vi "Configure Measurement.vi"(0 "VISA resource name":refnum<visa-resource-name>, 1 "Channel (1: Channel 1)":u16(ring)=1 items=["Channel 1"=1, "Channel 2"=2], 2 "Integration Time (4: 10 NPLCs)":u16(ring)=4 format="%.0g" items=["0.02 NPLC", "0.2 NPLC", "1 NPLC", "2 NPLCs", "10 NPLCs", "20 NPLCs", "100 NPLCs", "200 NPLCs"], 5 "Function (0: DC Volts)":u16(ring) items=["DC Volts", "DC Voltage Ratio", "DC Voltage Difference", "2 Wire Resistance", "4 Wire Resistance", "Temperature"], 7 "Auto Range (T:Enable)":bool=TRUE, 9 "Enable Offset Compensation (F: Disable)":bool, 11 "error in (no error)":errorcluster, 12 "Manual Range (0.001)":dbl=0.001, 13 "Resolution (1E-9)":dbl=1e-09 format="%^#_6g") -> (4 "VISA resource name out":refnum<visa-resource-name>, 15 "error out":errorcluster)   [LabVIEW 2022 SP3, in "Agilent 34420.lvlib"]
doc: "Configures the measurement type, resolution, and range on the instrument.\n\n<B>Note:</B>\n\nFor temperature measurements, further configuration is required. <B>Configure Temperature</B> VI should be called after this VI."
uses:
  Agilent 34420.lvlib
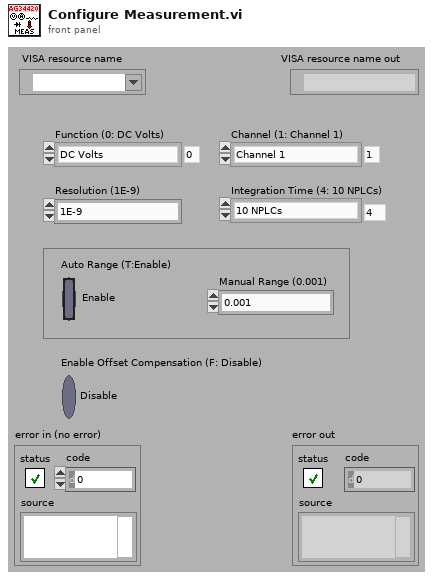
[diagram p1: front panel]
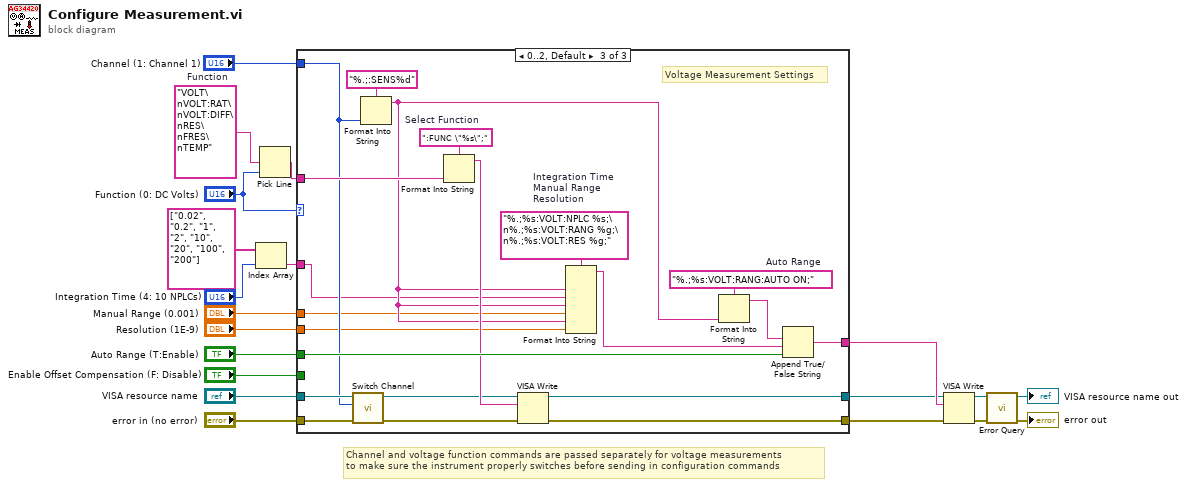
[diagram p0: block diagram]
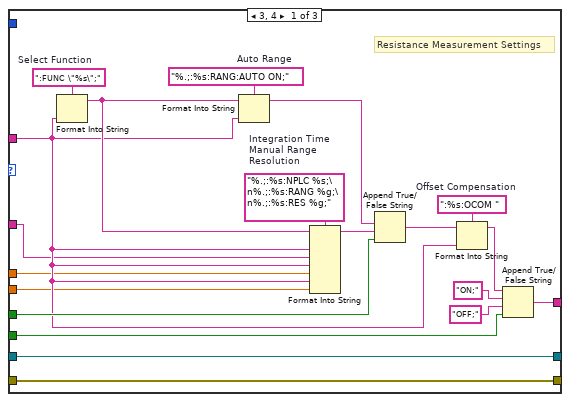
[diagram p2: hidden frame]
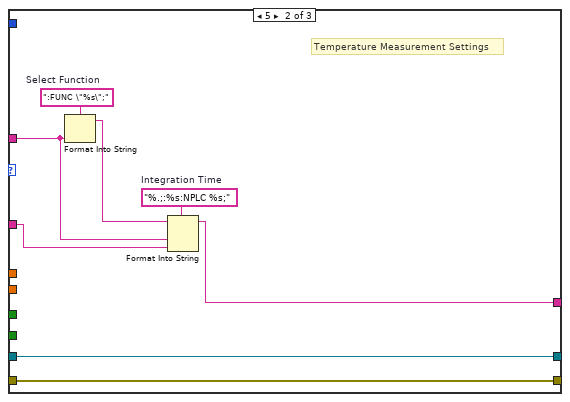
[diagram p3: hidden frame]
diagram:
  w18 = "VOLT\nVOLT:RAT\nVOLT:DIFF\nRES\nFRES\nTEMP"  # Function
  # "Channel and voltage function commands are passed separately for voltage measurements\nto make sure the instrument properly switches before sending in configuration commands"
  n1 = Index Array(array=string[] ["0.02", "0.2", "1", "2", "10", "20", "100", "200"], index="Integration Time (4: 10 NPLCs)") -> (element=w3:string)
  n2 = Pick Line(multi-line string=w18, line index="Function (0: DC Volts)") -> (output string=w15:string)  [unwired: 1 in]
  n3 = case shown="0..2, Default" "Function (0: DC Volts)" {
    tunnel: w15 -> [w24 w42 w65]
    tunnel: "Auto Range (T:Enable)" -> [w26 _ w64]
    tunnel: [w27 w48 w62] -> w13
    tunnel: "VISA resource name" -> [w29 w47 w61]
    tunnel: "error in (no error)" -> [w28 w46 w60]
    tunnel: "Channel (1: Channel 1)" -> [_ _ w59]
    tunnel: [w29 w47 w55] -> w9
    tunnel: [w28 w46 w54] -> w8
    tunnel: "Enable Offset Compensation (F: Disable)" -> [w25 _ _]
    tunnel: "Resolution (1E-9)" -> [w23 _ w50]
    tunnel: "Manual Range (0.001)" -> [w22 _ w51]
    tunnel: w3 -> [w21 w41 w49]
    frame 3, 4 {
      w34 = "%.;:%s:RANG:AUTO ON;"  # Auto Range
      w32 = "%.;:%s:NPLC %s;\n%.;:%s:RANG %g;\n%.;:%s:RES %g;"  # Integration Time Manual Range Resolution
      w31 = ":%s:OCOM "  # Offset Compensation
      w30 = ":FUNC \"%s\";"  # Select Function
      # "Resistance Measurement Settings"
      n4 = Format Into String(format string=w30, w24) -> (resulting string=w36:string)  [unwired: 2 in, 1 out]
      n5 = Format Into String(format string=w34, initial string=w36, w24) -> (resulting string=w35:string)  [unwired: 1 in, 1 out]
      n6 = Format Into String(format string=w32, initial string=w36, w24, w21, w24, w22, w24, w23) -> (resulting string=w33:string)  [unwired: 1 in, 1 out]
      n7 = Append True/False String(1:w26, 2:w33, 3:w35) -> (0:w37:string)  [unwired: 1 in]
      n8 = Format Into String(format string=w31, initial string=w37, w24) -> (resulting string=w38:string)  [unwired: 1 in, 1 out]
      n9 = Append True/False String(1:w25, 2:"OFF;" ("false string"), 3:"ON;" ("true string"), 4:w38) -> (0:w27:string)
    }
    frame 5 {
      w44 = ":FUNC \"%s\";"  # Select Function
      w45 = "%.;:%s:NPLC %s;"  # Integration Time
      # "Temperature Measurement Settings"
      n10 = Format Into String(format string=w44, w42) -> (resulting string=w43:string)  [unwired: 2 in, 1 out]
      n11 = Format Into String(format string=w45, initial string=w43, w42, w41) -> (resulting string=w48:string)  [unwired: 1 in, 1 out]
    }
    frame 0..2, Default {
      w67 = "%.;%s:VOLT:RANG:AUTO ON;"  # Auto Range
      w68 = "%.;%s:VOLT:NPLC %s;\n%.;%s:VOLT:RANG %g;\n%.;%s:VOLT:RES %g;"  # Integration Time Manual Range Resolution
      w69 = ":FUNC \"%s\";"  # Select Function
      # "Voltage Measurement Settings"
      n12 = call "Switch Channel.vi"("error in (no error)"=w60, "Channel (1: Channel 1)"=w59, "VISA resource name"=w61) -> ("error out"=w57:errorcluster, "VISA resource name out"=w56:refnum<visa-resource-name>)  [unwired: 7 in]
      n13 = Format Into String(format string="%.;:SENS%d", w59) -> (resulting string=w52:string)  [unwired: 2 in, 1 out]
      n14 = Format Into String(format string=w69, w65) -> (resulting string=w58:string)  [unwired: 2 in, 1 out]
      n15 = VISA Write(VISA resource name=w56, write buffer=w58, error in (no error)=w57) -> (VISA resource name out=w55:refnum<visa-resource-name>, error out=w54:errorcluster)  [unwired: 1 out]
      n16 = Format Into String(format string=w68, w52, w49, w52, w51, w52, w50) -> (resulting string=w53:string)  [unwired: 2 in, 1 out]
      n17 = Format Into String(format string=w67, w52) -> (resulting string=w66:string)  [unwired: 2 in, 1 out]
      n18 = Append True/False String(1:w64, 2:w53, 3:w66) -> (0:w62:string)  [unwired: 1 in]
    }
  }
  n19 = VISA Write(VISA resource name=w9, write buffer=w13, error in (no error)=w8) -> (VISA resource name out=w17:refnum<visa-resource-name>, error out=w16:errorcluster)  [unwired: 1 out]
  n20 = call "Error Query.vi"("error in (no error)"=w16, "VISA resource name"=w17) -> ("error out"=→"error out":errorcluster, "VISA resource name out"=→"VISA resource name out":refnum<visa-resource-name>)  [unwired: 6 in, 2 out]
